vi "Notebook.vi"() -> ()   [LabVIEW 2021, in "Notebook.lvlib"]
uses:
  Notebook.lvlib
  Notebook Action Q Element.ctl
  Notebook Action List.ctl
  Notebook Parameters List.ctl
  Rich Text Box/Formatted Text.ctl
  Rich Text Box/Text Formatting.ctl
  Rich Text Box/Text Colors.ctl
  Rich Text Box/Text Style.ctl
  Rich Text Box/Text Alignment.ctl
  Notebook Theme Edit Result.ctl
  Rich Text Box/Text Format List.ctl
  GUI/3-Button Dialog Output.ctl
  Variant/Variant to Data/Variant to Boolean.vi
  Variant/Variant to Data/Variant to Path.vi
  Variant/Variant to Data/Variant to String.vi
  System.Drawing
  Rich Text Box/Rich Text Box.lvlib
  System.Windows.Forms
  Variant/Variant to Data/Variant to Data.lvlib
  Strings/Strings.lvlib
  Error/Error.lvlib
  Utilities/Utilities.lvlib
  Fits/Fits.lvlib
panel:
  in  "Text Example":refnum<k24>(container) caption="Notebook Content"
  out "Notebook Updated":bool
  out "Message":string
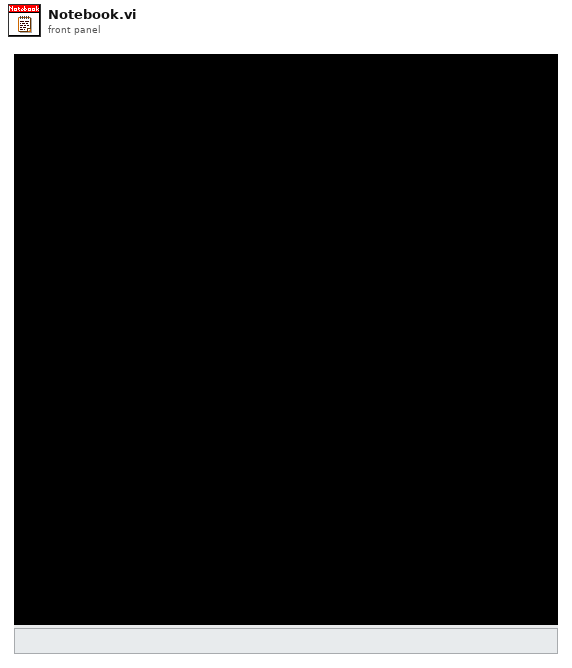
[diagram p1: front panel]
types:
  T1 = typedef "Notebook.lvlib/Notebook Parameters List.ctl" = enum16{"First Opening?", "Saved Notebook?", "Saved Notebook Path", "Beep on Error?", "Notebook Themes", "Current Theme Name"}
  T2 = enum32{"Invalid", "Standard", "Closed", "Hidden", "Minimized", "Maximized"}
  T3 = typedef "Notebook.lvlib/Notebook Action Q Element.ctl" = cluster{"Action":T4, "Variant":variant}
  T4 = typedef "Notebook.lvlib/Notebook Action List.ctl" = enum16{"Idle", "Init", "Check Content Change", "User added content", "Program added text", "Program added Picture ", "Save Notebook", "Quit", "Open", "Close", "Update Window Title", "Edit Text Styles", "Update Theme", "Save Themes", "Load Themes"}
  T5 = typedef "Rich Text Box.lvlib/Formatted Text.ctl" = cluster{"Text":string, "Text Formatting":T6}
  T6 = typedef "Rich Text Box.lvlib/Text Formatting.ctl" = cluster{"Font":string, "Text Color":T7, "Background Color":T7, "Style":T8, "Font Size":dbl, "Alignment":T9}
  T7 = typedef "Rich Text Box.lvlib/Text Colors.ctl" = enum16{"Unchanged", "Black", "Blue", "Cyan", "Maroon", "Gray", "Violet", "Green", "Light Green", "Orange", "Yellow", "Magenta", "Red", "White"}
  T8 = typedef "Rich Text Box.lvlib/Text Style.ctl" = enum16{"Regular", "Bold", "Italic", "Underline", "Strikeout"}
  T9 = typedef "Rich Text Box.lvlib/Text Alignment.ctl" = enum16{"Left", "Right", "Center"}
  T10 = typedef "Notebook.lvlib/Notebook Theme Edit Result.ctl" = enum16{"Cancelled", "Modified Theme", "New Theme", "Remove Theme"}
  T11 = typedef "Notebook.lvlib/Text Format List.ctl" = enum16{"Message", "Result", "Error", "Setting", "Verbose", "Warning"}
  T12 = typedef "Fits.lvlib/3-Button Dialog Output.ctl" = enum16{"Window Close", "Button 1", "Button 2", "Button 3"}
  T13 = typedef "Notebook.lvlib/Notebook Theme.ctl" = cluster{"Theme Name":string, "[Named Text Styles]":T14[], "Page Color":T7}
  T14 = typedef "Notebook.lvlib/Named Text Style.ctl" = cluster{"Text Formatting":T6, "Text Style Name":string}
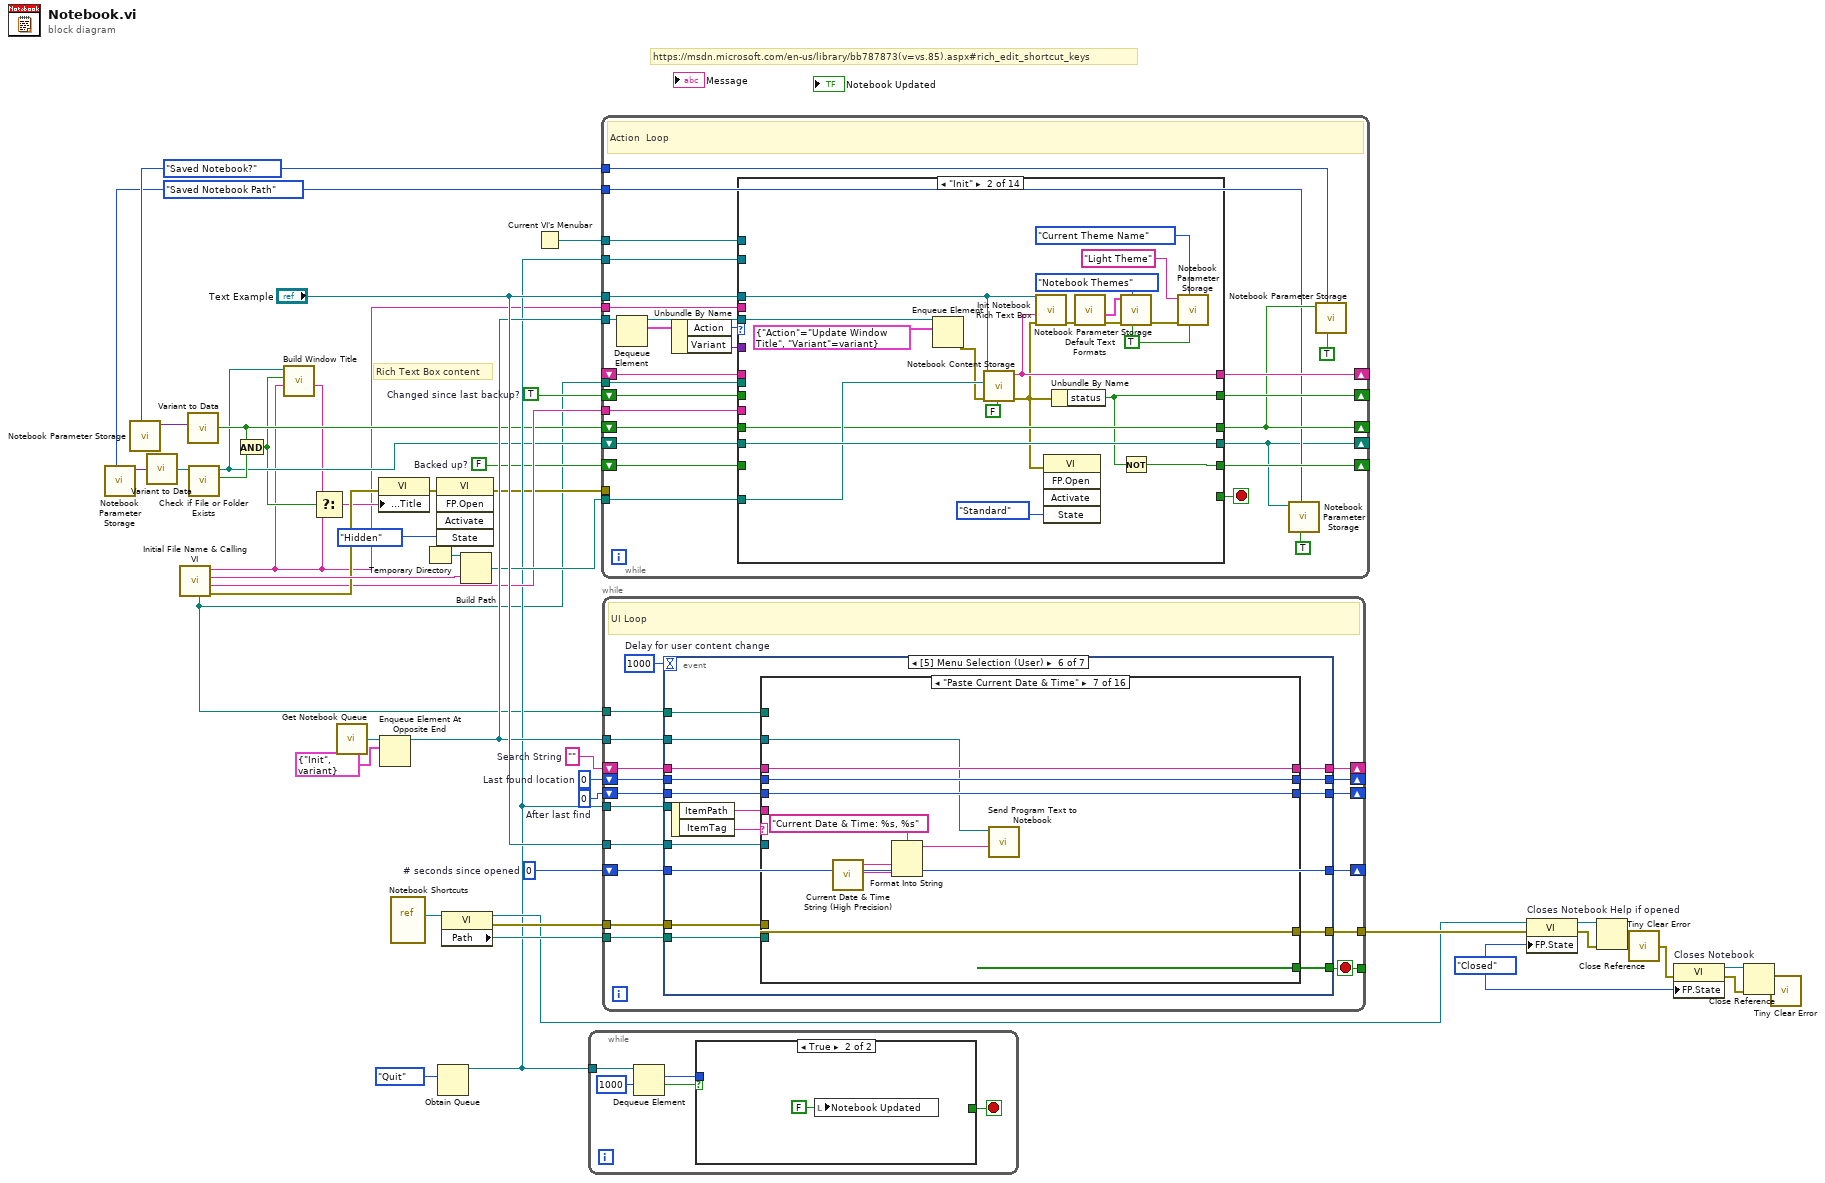
[diagram p0: block diagram]
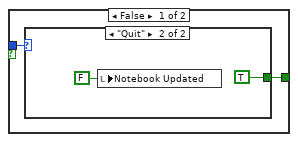
[diagram p2: hidden frame]
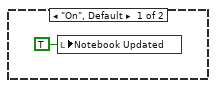
[diagram p3: hidden frame]
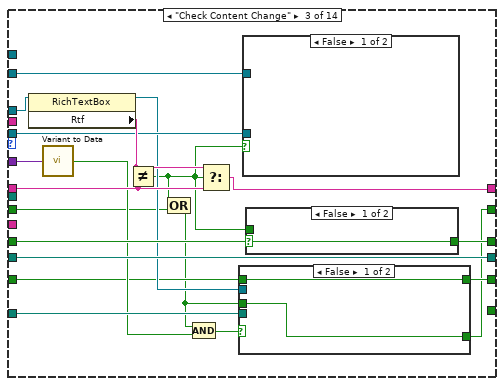
[diagram p5: hidden frame]
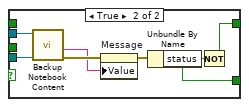
[diagram p6: hidden frame]
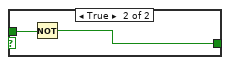
[diagram p7: hidden frame]
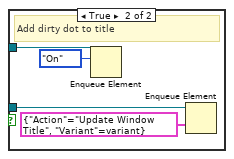
[diagram p8: hidden frame]
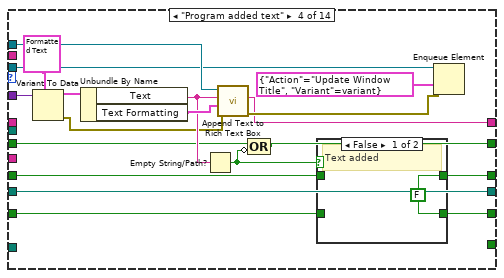
[diagram p9: hidden frame]
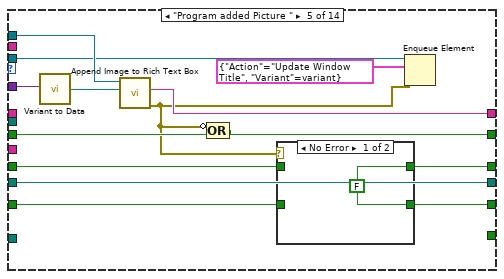
[diagram p11: hidden frame]
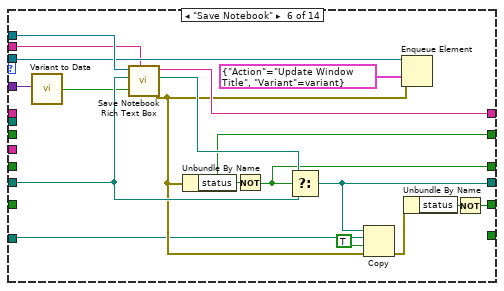
[diagram p13: hidden frame]
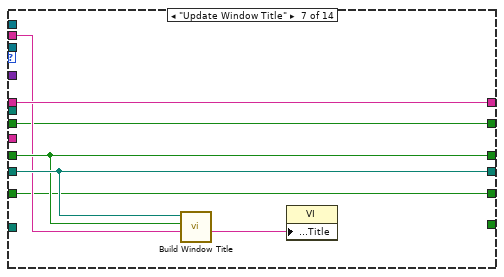
[diagram p14: hidden frame]
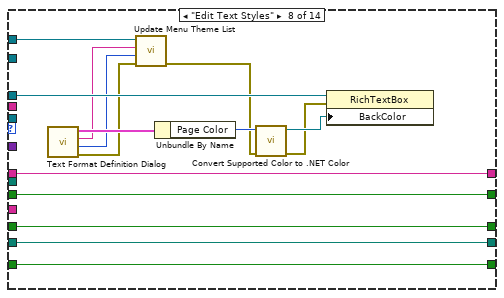
[diagram p15: hidden frame]
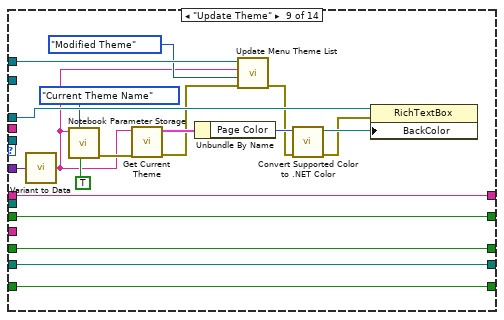
[diagram p16: hidden frame]
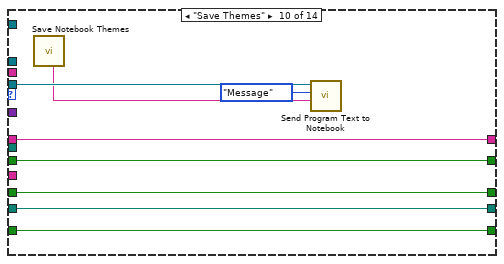
[diagram p17: hidden frame]
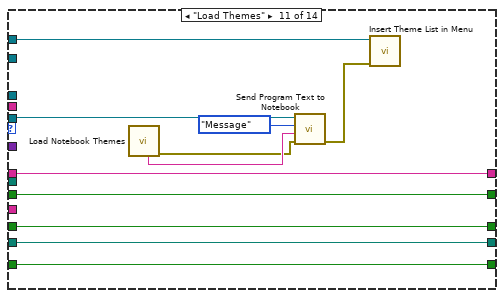
[diagram p18: hidden frame]
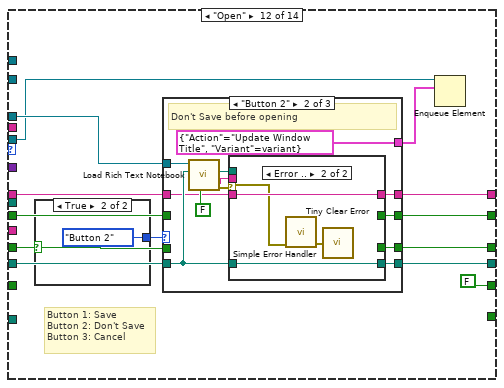
[diagram p19: hidden frame]
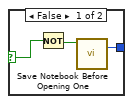
[diagram p20: hidden frame]
diagram:
  w11 = 0  # Last found location
  w12 = ""  # Search String
  w13 = 0  # After last find
  w14 = Notebook_Parameters_List."Saved Notebook Path" ("Notebook Parameter List")
  w15 = Notebook_Parameters_List."Saved Notebook?" ("Notebook Parameter List")
  w20 = TRUE  # Changed since last backup?
  w21 = FALSE  # Backed up?
  w22 = u64 0  # # seconds since opened
  w18 = T2."Closed" ("Front Panel Window:State")
  # "Rich Text Box content"
  # "https://msdn.microsoft.com/en-us/library/bb787873(v=vs.85).aspx#rich_edit_shortcut_keys"
  n1 = call "Notebook Parameter Storage.vi"("Notebook Parameter List"=w14) -> ("Data out"=w16:variant)  [unwired: 9 in, 1 out]
  n2 = call "Notebook Parameter Storage.vi"("Notebook Parameter List"=w15) -> ("Data out"=w17:variant)  [unwired: 9 in, 1 out]
  n3 = call-poly "Variant to Data.vi"("Variant"=w16) -> ("Path"=w10:path)  [unwired: 8 in]
  n4 = call "Initial File Name & Calling VI.vi"() -> ("error out"=w26:errorcluster, "Calling VI Name"=w25:string, "Backup File Name"=w40:string, "Default File Name"=w3:string, "Calling VI Path"=w2:path)  [unwired: 7 in]
  n5 = call-poly "Variant to Data.vi"("Variant"=w17) -> ("Value"=w9:bool)  [unwired: 8 in]
  n6 = call <vilib>:"Check if File or Folder Exists.vi"("path"=w10) -> ("file or folder exists?"=w8:bool, "dup path"=w6:path)  [unwired: 8 in, 1 out]
  n7 = And(x=w9, y=w8) -> (x .and. y?=w5:bool)
  n8 = call "Build Window Title.vi"("Root Window Title"=w3, "Saved Notebook?"=w5, "File Path in"=w6) -> ("Modified Window Title"=w4:string)  [unwired: 8 in]
  n9 = Select(t=w4, s=w5, f=w3) -> (s? t:f=w7:string)
  n10 = call "Get Notebook Queue.vi"() -> ("Notebook Queue"=w43:refnum<queue>)  [unwired: 9 in]
  n11 = property class="VI"(error in=w26, "Front Panel.Title"=w7) -> (error out=w38:errorcluster)  [unwired: 1 in, 1 out]
  n12 = Enqueue Element At Opposite End(queue=w43, element=T3 {"Action"=enum."Init", "Variant"=variant}) -> (queue out=w42:refnum<queue>)  [unwired: 2 in, 2 out]
  n13 = vi-ref "Notebook Shortcuts.vi"() -> (w35:refnum<vi>)
  n14 = Temporary Directory() -> (w45:path)
  n15 = invoke class="VI" method="FP.Open"(error in=w38, "State"=T2."Hidden") -> (error out=w19:errorcluster)  [unwired: 3 in, 4 out]
  n16 = Obtain Queue(element data type=enum16{"On", "Quit"}."Quit") -> (queue out=w23:refnum<queue>)  [unwired: 4 in, 2 out]
  n17 = property class="VI"(reference=w35) -> (reference out=w29:refnum<vi>, error out=w34:errorcluster, "Path"=w33:path)  [unwired: 1 in]
  n18 = Build Path(base path=w45, name or relative path=w40) -> (appended path=w39:path)
  n19 = Current VI's Menubar() -> (w1:refnum<k9>)
  n20 = while {
    tunnel: w23 -> [w52]
    stop <- w49 stop-if-true
    n21 = Dequeue Element(queue=w52, timeout in ms (-1)=1000) -> (element=w51:enum16{"On", "Quit"}, timed out?=w48:bool)  [unwired: 1 in, 2 out]
    n22 = case shown="True" w48 {
      tunnel: w51 -> [w54 _]
      tunnel: [w53 _] -> w49
      frame False {
        n23 = case shown="\"Quit\"" w54 {
          tunnel: [_ TRUE] -> w53
          frame "On", Default {
            n24 = local write "Notebook Updated"(TRUE ("Boolean Rectangle")) -> ()
          }
          frame "Quit" {
            n25 = local write "Notebook Updated"(FALSE ("Boolean Rectangle")) -> ()
          }
        }
      }
      frame True {
        n26 = local write "Notebook Updated"(FALSE ("Boolean Rectangle")) -> ()
      }
    }
  }
  n27 = while {
    tunnel: w42 -> [w85]
    shift-right: [w65] -> _
    shift-left: w9 -> [w82]
    shift-right: [w62] -> _
    shift-left: w6 -> [w81]
    tunnel: "Text Example" -> [w78]
    tunnel: w25 -> [w76]
    shift-right: [w75] -> _
    shift-left: _ -> [w74]
    tunnel: w39 -> [w73]
    tunnel: w3 -> [w72]
    tunnel: w23 -> [w71]
    shift-right: [w69] -> _
    shift-left: w21 -> [w70]
    shift-right: [w67] -> _
    shift-left: w20 -> [w68]
    tunnel: w19 -> [_]
    tunnel: w15 -> [w66]
    tunnel: w14 -> [w63]
    tunnel: w2 -> [w60]
    tunnel: w1 -> [w59]
    stop <- w77 stop-if-true
    # "Action  Loop"
    n28 = Dequeue Element(queue=w85) -> (queue out=w80:refnum<queue>, element=w84:T3)  [unwired: 2 in, 2 out]
    n29 = Unbundle By Name(w84) -> ("Action"=w83:T4, "Variant"=w79:variant)
    n30 = case shown="\"Init\"" w83 {
      tunnel: w82 -> [w90 w103 w125 w154 w174 _ w209 w226 w245 w253 w264 w271 w321 w327]
      tunnel: [w90 w103 w126 w153 w179 w195 w209 w226 w245 w253 w264 w275 w321 w327] -> w65
      tunnel: w81 -> [w89 w110 w131 w166 w183 w203 w211 w225 w244 w252 w263 w277 w322 w328]
      tunnel: [w89 w110 w131 w166 w183 w193 w211 w225 w244 w252 w263 w276 w322 w328] -> w62
      tunnel: w80 -> [_ w105 w127 w156 w177 w202 _ _ _ w248 w254 w273 w324 _]
      tunnel: w79 -> [_ _ w121 w164 w181 w200 _ _ w239 _ _ _ _ _]
      tunnel: w78 -> [_ w106 w122 w165 w182 w204 _ w221 w240 _ _ w274 w320 w338]
      tunnel: [_ _ _ _ _ _ _ _ _ _ _ _ w315 TRUE] -> w77
      tunnel: w76 -> [_ _ _ _ _ _ _ _ _ _ _ _ _ _]
      tunnel: [w88 w109 w128 w155 w176 w196 w208 w224 w243 w251 w262 w272 w323 ""] -> w75
      tunnel: w74 -> [w88 _ w129 _ _ _ w208 w224 w243 w251 w262 w269 w323 _]
      tunnel: w73 -> [_ w107 w123 _ _ w192 _ _ _ _ _ _ w319 w337]
      tunnel: w72 -> [_ _ _ _ _ w197 w207 _ _ _ _ _ _ _]
      tunnel: w71 -> [_ _ w119 _ _ _ _ _ _ _ _ _ w316 w334]
      tunnel: w70 -> [w87 _ w116 w152 w173 _ w206 w222 w241 w250 w261 _ _ _]
      tunnel: [w87 w102 w117 w151 w175 w188 w206 w222 w241 w250 w261 FALSE ("Backed up?") w312 w330] -> w69
      tunnel: w68 -> [w86 _ w114 w150 w172 _ w205 w223 w242 w249 w260 w265 w311 _]
      tunnel: [w86 w101 w113 w148 w170 w187 w205 w223 w242 w249 w260 w266 w311 FALSE ("Changed?")] -> w67
      tunnel: w60 -> [_ _ _ _ _ _ _ _ _ _ _ _ w310 _]
      tunnel: w59 -> [_ _ _ _ _ _ _ w216 w231 _ w259 _ _ _]
      frame "Idle", Default {
      }
      frame "Init" {
        w91 = TRUE ("Get(F)/Set")
        n31 = Enqueue Element(queue=w105, element=T3 {"Action"=enum."Update Window Title", "Variant"=variant}) -> (error out=w99:errorcluster)  [unwired: 2 in, 2 out]
        n32 = call "Notebook Content Storage.vi"("Save(T)/Load(F)"=FALSE ("Set(T)/Get(F)"), "Error In"=w99, "path"=w107, ".NET Refnum in"=w106) -> ("Error Out"=w100:errorcluster, "RTF content"=w109:string)  [unwired: 6 in]
        n33 = call "Init Notebook Rich Text Box.vi"("Error In"=w100, "Notebook Content"=w109, ".NET Refnum in"=w106) -> ("Error Out"=w98:errorcluster)  [unwired: 8 in]
        n34 = invoke class="VI" method="FP.Open"(error in=w100, "State"=T2."Standard") -> ()  [unwired: 3 in, 5 out]
        n35 = Unbundle By Name(w100) -> ("status"=w101:bool)
        n36 = call "Default Text Formats.vi"("Error In"=w98) -> ("Error Out"=w97:errorcluster, "Base Themes"=w96:T13[])  [unwired: 8 in, 1 out]
        n37 = call "Notebook Parameter Storage.vi"("Get(F)/Set"=w91, "Notebook Parameter List"=Notebook_Parameters_List."Notebook Themes", "Error In"=w97, "Data in"=w96) -> ("Error Out"=w94:errorcluster)  [unwired: 6 in, 1 out]
        n38 = Not(x=w101) -> (.not. x?=w102:bool)
        n39 = call "Notebook Parameter Storage.vi"("Get(F)/Set"=w91, "Notebook Parameter List"=Notebook_Parameters_List."Current Theme Name", "Error In"=w94, "Data in"="Light Theme" ("RTF content")) -> ()  [unwired: 6 in, 2 out]
      }
      frame "Check Content Change" {
        n40 = property class="RichTextBox"(reference=w122) -> (reference out=w124:refnum<k24>, "Rtf"=w130:string)  [unwired: 1 in, 1 out]
        n41 = call-poly "Variant to Data.vi"("Variant"=w121) -> ("Value"=w120:bool)  [unwired: 8 in]
        n42 = Not Equal?(x=w130, y=w129) -> (x != y?=w115:bool)
        n43 = Compound Arithmetic op=OR(w115, w114) -> (w112:bool)
        n44 = Compound Arithmetic op=AND(w112, w120) -> (w118:bool)
        n45 = Select(t=w130, s=w115, f=w129) -> (s? t:f=w128:string)
        n46 = case shown="False" w118 {
          tunnel: w124 -> [_ w140]
          tunnel: w123 -> [_ w138]
          tunnel: [w133 w135] -> w117
          tunnel: w116 -> [w133 _]
          tunnel: [w132 w134] -> w113
          tunnel: w112 -> [w132 _]
          frame False {
          }
          frame True {
            n47 = call "Backup Notebook Content.vi"("Notebook Backup Path"=w138, "Rich Text Box .NET Refnum"=w140) -> ("error out"=w139:errorcluster, "Message"=w137:string)  [unwired: 8 in]
            n48 = property on="Message" class="Str"(error in=w139, "Value"=w137) -> (error out=w136:errorcluster)  [unwired: 1 in, 1 out]
            n49 = Unbundle By Name(w136) -> ("status"=w134:bool)
            n50 = Not(x=w134) -> (.not. x?=w135:bool)
          }
        }
        n51 = case shown="False" w115 {
          tunnel: w127 -> [_ w147]
          tunnel: w119 -> [_ w145]
          frame False {
          }
          frame True {
            # "Add dirty dot to title"
            n52 = Enqueue Element(queue=w145, element=enum16{"On", "Quit"}."On") -> ()  [unwired: 2 in, 3 out]
            n53 = Enqueue Element(queue=w147, element=T3 {"Action"=enum."Update Window Title", "Variant"=variant}) -> ()  [unwired: 2 in, 3 out]
          }
        }
        n54 = case shown="False" w125 {
          selector: w125 -> [w141 _]
          tunnel: w115 -> [_ w143]
          tunnel: [w141 w142] -> w126
          frame False {
          }
          frame True {
            n55 = Not(x=w143) -> (.not. x?=w142:bool)
          }
        }
      }
      frame "Program added text" {
        n56 = Variant To Data(type=T5 {"Text"="", "Text Formatting"={"Font"="", "Text Color"=enum."Unchanged", "Background Color"=enum."Unchanged", "Style"=enum."Regular", "Font Size"=-1.0, "Alignment"=enum."Left"}} ("Formatted Text"), Variant=w164) -> (data=w162:T5, error out=w159:errorcluster)  [unwired: 1 in]
        n57 = Unbundle By Name(w162) -> ("Text"=w160:string, "Text Formatting"=w161:T6)
        n58 = Empty String/Path?(string/path=w160) -> (empty?=w149:bool)
        n59 = call "Append Text to Rich Text Box.vi"("error in (no error)"=w159, "Text Formatting"=w161, "String"=w160, ".NET Refnum in"=w165) -> ("Error Out"=w157:errorcluster, "Rtf Content"=w155:string)  [unwired: 5 in, 1 out]
        n60 = Compound Arithmetic op=OR(w150, invert w149) -> (w148:bool)
        n61 = case shown="False" w149 {
          tunnel: w154 -> [_ w169]
          tunnel: [w167 w169] -> w153
          tunnel: w152 -> [_ w168]
          tunnel: [w167 w168] -> w151
          frame False {
            w167 = FALSE ("Saved Notebook?")
            # "Text added"
          }
          frame True {
            # "No change"
          }
        }
        n62 = Enqueue Element(queue=w156, element=T3 {"Action"=enum."Update Window Title", "Variant"=variant}, error in (no error)=w157) -> ()  [unwired: 1 in, 3 out]
      }
      frame "Program added Picture " {
        n63 = call-poly "Variant to Data.vi"("Variant"=w181) -> ("Path"=w180:path)  [unwired: 8 in]
        n64 = call "Append Image to Rich Text Box.vi"("Image File Path"=w180, ".NET Refnum in"=w182) -> ("error out"=w171:errorcluster, "Rtf Content"=w176:string)  [unwired: 8 in]
        n65 = Compound Arithmetic op=OR(invert w171, w172) -> (w170:bool)
        n66 = case shown="No Error" w171 {
          tunnel: [w184 w186] -> w179
          tunnel: [w184 w185] -> w175
          tunnel: w174 -> [_ w186]
          tunnel: w173 -> [_ w185]
          frame No Error {
            w184 = FALSE ("Saved?")
          }
          frame Error {
          }
        }
        n67 = Enqueue Element(queue=w177, element=T3 {"Action"=enum."Update Window Title", "Variant"=variant}, error in (no error)=w171) -> ()  [unwired: 1 in, 3 out]
      }
      frame "Save Notebook" {
        n68 = call-poly "Variant to Data.vi"("Variant"=w200) -> ("Value"=w199:bool)  [unwired: 8 in]
        n69 = call "Save Notebook Rich Text Box.vi"("Default Notebook File Name (Notebook)"=w197, "Dialog (F)"=w199, "File Path Control"=w203, ".NET Refnum in"=w204) -> ("Error Out"=w194:errorcluster, "File Path out"=w198:path, "Rtf Content"=w196:string)  [unwired: 4 in, 1 out]
        n70 = Unbundle By Name(w194) -> ("status"=w187:bool)
        n71 = Not(x=w187) -> (.not. x?=w195:bool)
        n72 = Select(t=w198, s=w195, f=w203) -> (s? t:f=w193:path)
        n73 = Copy(8:w194, 9:TRUE ("overwrite (F)"), 10:w192, 11:w193) -> (0:w190:errorcluster)  [unwired: 1 in, 2 out]
        n74 = Enqueue Element(queue=w202, element=T3 {"Action"=enum."Update Window Title", "Variant"=variant}, error in (no error)=w194) -> ()  [unwired: 1 in, 3 out]
        n75 = Unbundle By Name(w190) -> ("status"=w189:bool)
        n76 = Not(x=w189) -> (.not. x?=w188:bool)
      }
      frame "Update Window Title" {
        n77 = call "Build Window Title.vi"("Root Window Title"=w207, "Saved Notebook?"=w209, "File Path in"=w211) -> ("Modified Window Title"=w210:string)  [unwired: 8 in]
        n78 = property class="VI"("Front Panel.Title"=w210) -> ()  [unwired: 2 in, 2 out]
      }
      frame "Edit Text Styles" {
        n79 = call "Text Format Definition Dialog.vi"() -> ("Error Out"=w213:errorcluster, "Result"=w215:T10, "Theme Name"=w214:string, "Notebook Theme"=w218:T13)  [unwired: 8 in]
        n80 = call "Update Menu Theme List.vi"("error in (no error)"=w213, "Result"=w215, "Theme Name"=w214, "Menu in"=w216) -> ("error out"=w212:errorcluster)  [unwired: 7 in]
        n81 = Unbundle By Name(w218) -> ("Page Color"=w217:T7)
        n82 = call "Convert Supported Color to .NET Color.vi"("error in (no error)"=w212, "Text Color"=w217) -> ("error out"=w219:errorcluster, ".NET Color"=w220:refnum<k24>)  [unwired: 8 in]
        n83 = property class="RichTextBox"(reference=w221, error in=w219, "BackColor"=w220) -> ()  [unwired: 2 out]
      }
      frame "Update Theme" {
        n84 = call-poly "Variant to Data.vi"("Variant"=w239) -> ("String"=w229:string)  [unwired: 8 in]
        n85 = call "Notebook Parameter Storage.vi"("Get(F)/Set"=TRUE, "Notebook Parameter List"=Notebook_Parameters_List."Current Theme Name", "Data in"=w229) -> ("Error Out"=w233:errorcluster)  [unwired: 7 in, 1 out]
        n86 = call "Get Current Theme.vi"("Error In"=w233, "Theme Name"=w229) -> ("Error Out"=w228:errorcluster, "Notebook Theme"=w232:T13)  [unwired: 7 in, 1 out]
        n87 = Unbundle By Name(w232) -> ("Page Color"=w236:T7)
        n88 = call "Update Menu Theme List.vi"("error in (no error)"=w228, "Result"=Notebook_Theme_Edit_Result."Modified Theme", "Theme Name"=w229, "Menu in"=w231) -> ("error out"=w227:errorcluster)  [unwired: 7 in]
        n89 = call "Convert Supported Color to .NET Color.vi"("error in (no error)"=w227, "Text Color"=w236) -> ("error out"=w237:errorcluster, ".NET Color"=w238:refnum<k24>)  [unwired: 8 in]
        n90 = property class="RichTextBox"(reference=w240, error in=w237, "BackColor"=w238) -> ()  [unwired: 2 out]
      }
      frame "Save Themes" {
        n91 = call "Save Notebook Themes.vi"() -> ("Message"=w247:string)  [unwired: 8 in, 3 out]
        n92 = call "Send Program Text to Notebook.vi"("Text (none)"=w247, "Text Format (Message)"=Text_Format_List."Message" ("Text Format"), "Notebook Queue in"=w248) -> ()  [unwired: 8 in, 1 out]
      }
      frame "Load Themes" {
        n93 = call "Load Notebook Themes.vi"() -> ("error out"=w256:errorcluster, "Message"=w257:string)  [unwired: 8 in, 2 out]
        n94 = call "Send Program Text to Notebook.vi"("Error In"=w256, "Text (none)"=w257, "Text Format (Message)"=Text_Format_List."Message" ("Text Format"), "Notebook Queue in"=w254) -> ("Error Out"=w255:errorcluster)  [unwired: 7 in]
        n95 = call "Insert Theme List in Menu.vi"("error in (no error)"=w255, "Menu in"=w259) -> ()  [unwired: 9 in, 1 out]
      }
      frame "Open" {
        # "Button 1: Save\nButton 2: Don't Save\nButton 3: Cancel"
        n96 = case shown="True" w271 {
          selector: w271 -> [w280 _]
          tunnel: [w279 3-Button_Dialog_Output."Button 2" ("Save/Don't Save/Cancel")] -> w270
          frame False {
            n97 = Not(x=w280) -> (.not. x?=w278:bool)
            n98 = call "Save Notebook Before Opening One.vi"("Not saved?"=w278) -> ("Save/Don't Save/Cancel"=w279:T12)  [unwired: 9 in, 1 out]
          }
          frame True {
          }
        }
        n99 = case shown="\"Button 2\"" w270 {
          tunnel: w277 -> [w285 w293 w308]
          tunnel: [w285 w298 w308] -> w276
          tunnel: [w286 w292 w307] -> w275
          tunnel: w271 -> [w286 _ w307]
          tunnel: w274 -> [_ w297 _]
          tunnel: [w284 w288 w309] -> w272
          tunnel: w269 -> [w284 w289 w309]
          tunnel: [T3 {"Action"=enum."Save Notebook", "Variant"=variant} ("element") T3 {"Action"=enum."Update Window Title", "Variant"=variant} ("element") _] -> w268
          tunnel: [w282 w287 w306] -> w266
          tunnel: w265 -> [w282 _ w306]
          frame "Button 1" {
            # "Save"
            # "Save"
          }
          frame "Button 2" {
            # "Don't Save before opening"
            n100 = call "Load Rich Text Notebook.vi"("Backup?"=FALSE, "File Path Control"=w293, ".NET Refnum in"=w297) -> ("Error Out"=w290:errorcluster, "File Path out"=w296:path, "RTF content"=w291:string)  [unwired: 4 in, 2 out]
            n101 = case shown="Error .." w290 {
              selector: w290 -> [_ w303]
              tunnel: [w301 w305] -> w298
              tunnel: w296 -> [w301 _]
              tunnel: w293 -> [_ w305]
              tunnel: [w299 _] -> w292
              tunnel: w291 -> [w300 _]
              tunnel: w289 -> [_ w304]
              tunnel: [w300 w304] -> w288
              tunnel: [w299 _] -> w287
              frame No Error {
                w299 = TRUE ("status")
              }
              frame Error {
                n102 = call <vilib>:"Simple Error Handler.vi"("error in (no error)"=w303) -> ("error out"=w302:errorcluster)  [unwired: 4 in, 4 out]
                n103 = call "Tiny Clear Error.vi"("Error In"=w302) -> ()  [unwired: 8 in, 1 out]
              }
            }
          }
          frame "Button 3", Default {
            # "Cancel"
          }
        }
        n104 = Enqueue Element(queue=w273, element=w268) -> ()  [unwired: 2 in, 3 out]
      }
      frame "Close" {
        n105 = call "Close Notebook Window Action.vi"("Notebook Saved?"=w321, "Main VI Path"=w310, "Notebook Queue"=w324) -> ("Quit?"=w315:bool)  [unwired: 8 in]
        n106 = call "Backup Notebook Content.vi"("Notebook Backup Path"=w319, "Rich Text Box .NET Refnum"=w320) -> ("error out"=w317:errorcluster, "Message"=w318:string)  [unwired: 8 in]
        n107 = case shown="True" w315 {
          tunnel: w316 -> [_ w325]
          frame False {
          }
          frame True {
            n108 = Enqueue Element(queue=w325, element=enum16{"On", "Quit"}."Quit") -> ()  [unwired: 2 in, 3 out]
          }
        }
        n109 = property on="Message" class="Str"(error in=w317, "Value"=w318) -> (error out=w314:errorcluster)  [unwired: 1 in, 1 out]
        n110 = Unbundle By Name(w314) -> ("status"=w313:bool)
        n111 = Not(x=w313) -> (.not. x?=w312:bool)
      }
      frame "Quit" {
        n112 = Enqueue Element(queue=w334, element=enum16{"On", "Quit"}."Quit") -> ()  [unwired: 2 in, 3 out]
        n113 = call "Backup Notebook Content.vi"("Notebook Backup Path"=w337, "Rich Text Box .NET Refnum"=w338) -> ("error out"=w335:errorcluster, "Message"=w336:string)  [unwired: 8 in]
        n114 = property on="Message" class="Str"(error in=w335, "Value"=w336) -> (error out=w332:errorcluster)  [unwired: 1 in, 1 out]
        n115 = Unbundle By Name(w332) -> ("status"=w331:bool)
        n116 = Not(x=w331) -> (.not. x?=w330:bool)
      }
    }
    n117 = call "Notebook Parameter Storage.vi"("Get(F)/Set"=TRUE, "Notebook Parameter List"=w63, "Data in"=w62) -> ()  [unwired: 7 in, 2 out]
    n118 = call "Notebook Parameter Storage.vi"("Get(F)/Set"=TRUE, "Notebook Parameter List"=w66, "Data in"=w65) -> ()  [unwired: 7 in, 2 out]
  }
  n119 = while {
    tunnel: w42 -> [w357]
    tunnel: "Text Example" -> [w355]
    tunnel: w34 -> [w354]
    tunnel: w33 -> [w353]
    tunnel: [w352] -> _
    tunnel: [w351] -> w30
    tunnel: w23 -> [w350]
    shift-right: [w348] -> _
    shift-left: w22 -> [w349]
    shift-right: [w347] -> _
    shift-left: w13 -> [w344]
    shift-right: [w346] -> _
    shift-left: w12 -> [w345]
    shift-right: [w342] -> _
    shift-left: w11 -> [w343]
    tunnel: w2 -> [w341]
    stop <- w352 stop-if-true
    w356 = 1000  # Delay for user content change
    # "UI Loop"
    n120 = event shown="[5] Menu Selection (User)" {
      selector: _ -> [_ _ _ _ _ _ _]
      dyn-events: _ -> [_ _ _ _ _ _ _]
      timeout: w356 -> [_ _ _ _ _ _ _]
      tunnel: [w366 _ _ _ _ w493 _] -> w352
      tunnel: w357 -> [w368 w374 w455 _ w479 w494 _]
      tunnel: w355 -> [_ w378 _ w463 _ w488 w636]
      tunnel: w341 -> [w358 _ _ _ _ w481 _]
      tunnel: w354 -> [_ _ _ _ _ w492 _]
      tunnel: w353 -> [_ _ _ _ _ w491 _]
      tunnel: [_ _ _ _ _ w490 _] -> w351
      tunnel: w350 -> [_ w373 _ _ _ _ _]
      tunnel: w349 -> [w365 w372 w454 w465 w476 w489 w635]
      tunnel: [w365 w372 w454 w465 w474 w489 w635] -> w348
      tunnel: [w360 w370 w452 w458 w470 w487 w633] -> w347
      tunnel: [w361 w371 w453 w459 w471 w486 w634] -> w346
      tunnel: w345 -> [w361 w371 w453 w459 w471 w485 w634]
      tunnel: w344 -> [w360 w370 w452 w458 w470 w484 w633]
      tunnel: w343 -> [w359 w369 w451 w457 w469 w482 w632]
      tunnel: [w359 w369 w451 w457 w469 w483 w632] -> w342
      event Panel Close? {
        n121 = event-data() -> ()  [unwired: 1 in, 1 out]
        n122 = call "Notebook Parameter Storage.vi"("Notebook Parameter List"=Notebook_Parameters_List."Saved Notebook?") -> ("Data out"=w364:variant)  [unwired: 9 in, 1 out]
        n123 = call-poly "Variant to Data.vi"("Variant"=w364) -> ("Value"=w362:bool)  [unwired: 8 in]
        n124 = call "Close Notebook Window Action.vi"("Notebook Saved?"=w362, "Main VI Path"=w358, "Notebook Queue"=w368) -> ("Quit?"=w366:bool)  [unwired: 8 in]
        n125 = event-data("Discard?"=TRUE) -> ()  [unwired: 1 in, 1 out]
      }
      event "Text Example": Shortcut Menu Selection (User) {
        n126 = event-data() -> ("ItemTag"=w379:string)  [unwired: 1 in]
        n127 = property class="RichTextBox"(reference=w378) -> (reference out=w375:refnum<k24>, error out=w376:errorcluster, "SelectionFont"=w377:refnum<k24>)  [unwired: 1 in]
        n128 = case shown="\"B_Black\", \"B_Blue\", \"B_Cyan\", \"B_Gray\", \"B_Green\", \"B_Light Green\", \"B_Magenta\", \"B_Maroon\", \"B_Orange\", \"B_Red\", \"B_Violet\", \"B_White\", \"B_Yellow\"" w379 {
          selector: w379 -> [_ w390 w397 w411 w432]
          tunnel: w377 -> [_ w384 w401 _ _]
          tunnel: w376 -> [_ w383 w396 w412 w434]
          tunnel: w375 -> [_ w380 w393 w413 w435]
          tunnel: w374 -> [_ _ _ _ _]
          tunnel: w373 -> [_ _ w391 w409 w433]
          frame "" {
          }
          frame "5 pt", Default {
            n129 = property class="Font"(reference=w384, error in=w383) -> (error out=w387:errorcluster, "Name"=w388:string, "Style"=w382:i32)  [unwired: 1 out]
            n130 = Scan From String(format string="%d pt", input string=w390) -> (output 1=w381:i32)  [unwired: 3 in, 3 out]
            n131 = constructor class="Font"(error in=w387, "familyName"=w388, "emSize"=w381, "unit"=w382) -> (reference out=w385:refnum<k24>, error out=w386:errorcluster)  [unwired: 2 in, 4 out]
            n132 = property class="RichTextBox"(reference=w380, error in=w386, "SelectionFont"=w385) -> ()  [unwired: 2 out]
          }
          frame "Bold", "Italic", "Regular", "Strikeout", "Underline" {
            n133 = disable-structure shown="Disabled" {
              disable-tunnel: w391 -> [w402 _]
              frame Disabled {
                n134 = Enqueue Element(queue=w402, element=enum16{"On", "Quit"}."On") -> ()  [unwired: 2 in, 3 out]
              }
              frame Enabled {
              }
            }
            n135 = property class="Font"(reference=w401, error in=w396) -> (error out=w395:errorcluster, "Name"=w400:string, "SizeInPoints"=w399:sgl)  [unwired: 1 out]
            n136 = case shown="\"Bold\"" w397 {
              tunnel: [w404 w405 w406 w407 w408] -> w398
              frame "Regular", Default {
                w404 = 0 items=["Regular"=0, "Bold"=1, "Italic"=2, "Underline"=4, "Strikeout"=8] ("style")
              }
              frame "Bold" {
                w405 = 1 items=["Regular"=0, "Bold"=1, "Italic"=2, "Underline"=4, "Strikeout"=8] ("style")
              }
              frame "Italic" {
                w406 = 2 items=["Regular"=0, "Bold"=1, "Italic"=2, "Underline"=4, "Strikeout"=8] ("style")
              }
              frame "Underline" {
                w407 = 4 items=["Regular"=0, "Bold"=1, "Italic"=2, "Underline"=4, "Strikeout"=8] ("style")
              }
              frame "Strikeout" {
                w408 = 8 items=["Regular"=0, "Bold"=1, "Italic"=2, "Underline"=4, "Strikeout"=8] ("style")
              }
            }
            n137 = constructor class="Font"(error in=w395, "familyName"=w400, "emSize"=w399, "unit"=w398) -> (reference out=w392:refnum<k24>, error out=w394:errorcluster)  [unwired: 2 in, 4 out]
            n138 = property class="RichTextBox"(reference=w393, error in=w394, "SelectionFont"=w392) -> ()  [unwired: 2 out]
          }
          frame "Black", "Blue", "Cyan", "Gray", "Green", "Light Green", "Magenta", "Maroon", "Orange", "Red", "Violet", "White", "Yellow" {
            n139 = case shown="\"Orange\"" w411 {
              tunnel: [Text_Colors."Black" ("Text Color") Text_Colors."Blue" ("Text Color") Text_Colors."Cyan" ("Text Color") Text_Colors."Gray" ("Text Color") Text_Colors."Green" ("Text Color") Text_Colors."Light Green" ("Text Color") Text_Colors."Magenta" ("Text Color") Text_Colors."Maroon" ("Text Color") Text_Colors."Orange" ("Text Color") Text_Colors."Red" ("Text Color") Text_Colors."Violet" ("Text Color") Text_Colors."White" ("Text Color") Text_Colors."Yellow" ("Text Color")] -> w410
              frame "Black", Default {
              }
              frame "Blue" {
              }
              frame "Cyan" {
              }
              frame "Gray" {
              }
              frame "Green" {
              }
              frame "Light Green" {
              }
              frame "Magenta" {
              }
              frame "Maroon" {
              }
              frame "Orange" {
              }
              frame "Red" {
              }
              frame "Violet" {
              }
              frame "White" {
              }
              frame "Yellow" {
              }
            }
            n140 = disable-structure shown="Disabled" {
              disable-tunnel: w409 -> [w414 _]
              frame Disabled {
                n141 = Enqueue Element(queue=w414, element=enum16{"On", "Quit"}."On") -> ()  [unwired: 2 in, 3 out]
              }
              frame Enabled {
              }
            }
            n142 = call "Set RTB Selection Text Color.vi"("Error In"=w412, "Text Color"=w410, ".NET RTB Refnum in"=w413) -> ()  [unwired: 7 in, 2 out]
          }
          frame "B_Black", "B_Blue", "B_Cyan", "B_Gray", "B_Green", "B_Light Green", "B_Magenta", "B_Maroon", "B_Orange", "B_Red", "B_Violet", "B_White", "B_Yellow" {
            n143 = disable-structure shown="Disabled" {
              disable-tunnel: w433 -> [w450 _]
              frame Disabled {
                n144 = Enqueue Element(queue=w450, element=enum16{"On", "Quit"}."On") -> ()  [unwired: 2 in, 3 out]
              }
              frame Enabled {
              }
            }
            n145 = String Subset(string=w432, offset (0)=2) -> (substring=w430:string)  [unwired: 1 in]
            n146 = case shown="\"Cyan\"" w430 {
              tunnel: [Text_Colors."Black" ("Text Color") Text_Colors."Blue" ("Text Color") Text_Colors."Cyan" ("Text Color") Text_Colors."Gray" ("Text Color") Text_Colors."Green" ("Text Color") Text_Colors."Light Green" ("Text Color") Text_Colors."Magenta" ("Text Color") Text_Colors."Maroon" ("Text Color") Text_Colors."Orange" ("Text Color") Text_Colors."Red" ("Text Color") Text_Colors."Violet" ("Text Color") Text_Colors."White" ("Text Color") Text_Colors."Yellow" ("Text Color")] -> w431
              frame "Black", Default {
              }
              frame "Blue" {
              }
              frame "Cyan" {
              }
              frame "Gray" {
              }
              frame "Green" {
              }
              frame "Light Green" {
              }
              frame "Magenta" {
              }
              frame "Maroon" {
              }
              frame "Orange" {
              }
              frame "Red" {
              }
              frame "Violet" {
              }
              frame "White" {
              }
              frame "Yellow" {
              }
            }
            n147 = call "Set RTB Selection Text Background Color.vi"("Error In"=w434, "Text Background Color"=w431, ".NET RTB Refnum in"=w435) -> ()  [unwired: 7 in, 2 out]
          }
        }
      }
      event "Text Example": Value Change {
        n148 = event-data() -> ()  [unwired: 1 in, 3 out]
        n149 = Enqueue Element(queue=w455, element=T3 {"Action"=enum."Check Content Change", "Variant"=variant}) -> ()  [unwired: 2 in, 3 out]
      }
      event "Text Example": Mouse Down? {
        n150 = event-data() -> ("Button"=w460:u16, "Coords.Horizontal"=w462:i32, "Coords.Vertical"=w461:i32)  [unwired: 1 in]
        n151 = case shown="1" w460 {
          tunnel: w463 -> [_ w468]
          tunnel: w462 -> [_ w467]
          tunnel: w461 -> [_ w466]
          frame 2, Default {
            # "right click"
          }
          frame 1 {
            # "Left Click"
            n152 = call "Set Cursor to Mouse Click.vi"("Vertical"=w466, "Horizontal"=w467, "RichTextBox Refnum"=w468) -> ()  [unwired: 8 in, 1 out]
          }
        }
        n153 = event-data("Discard?"=FALSE) -> ()  [unwired: 4 in, 1 out]
      }
      event Timeout {
        w475 = u64 300  # Delay for backup (x timeout)
        n154 = event-data() -> ()  [unwired: 1 in, 1 out]
        n155 = Increment(x=w476) -> (x+1=w474:u64)
        n156 = Quotient & Remainder(x=w474, y=w475) -> (x-y*floor(x/y)=w473:u64)  [unwired: 1 out]
        n157 = Equal To 0?(x=w473) -> (x = 0?=w472:bool)
        n158 = Bundle By Name(cluster=T3 {"Action"=enum."Check Content Change", "Variant"=variant} ("element"), "Variant"=w472) -> (w477:T3)
        n159 = Enqueue Element(queue=w479, element=w477) -> ()  [unwired: 2 in, 3 out]
      }
      event Menu Selection (User) {
        n160 = event-data() -> ("ItemPath"=w480:string, "ItemTag"=w495:string)  [unwired: 1 in]
        n161 = case shown="\"Paste Current Date & Time\"" w495 {
          selector: w495 -> [_ _ _ _ _ _ _ _ _ _ _ _ w603 w613 _ _]
          tunnel: w494 -> [_ w505 w513 w521 w531 _ w536 _ _ _ _ w594 w604 w615 _ _]
          tunnel: [_ _ _ _ w530 _ _ _ _ _ _ _ _ _ _ _] -> w493
          tunnel: w481 -> [_ _ _ _ w529 _ _ _ _ _ _ _ _ _ _ _]
          tunnel: w492 -> [w499 w503 w509 w517 w528 w535 w541 w550 w560 w580 w593 w599 w608 w619 w625 w630]
          tunnel: w491 -> [_ _ _ _ _ _ _ _ _ _ _ _ _ _ _ w631]
          tunnel: [w499 w503 w509 w517 w528 w535 w541 w548 w556 w572 w593 w599 w608 w619 w625 w629] -> w490
          tunnel: w488 -> [_ _ _ _ _ _ _ w549 w561 w581 _ _ _ _ _ _]
          tunnel: [w497 w501 w507 w515 w523 w533 w539 w546 w558 w573 w592 w598 w607 w618 w623 w627] -> w487
          tunnel: [w498 w502 w508 w516 w524 w534 w540 w547 w555 w571 w591 w597 w606 w617 w624 w628] -> w486
          tunnel: w485 -> [w498 w502 w508 w516 w524 w534 w540 _ w555 w571 w591 w597 w606 w617 w624 w628]
          tunnel: w484 -> [w497 w501 w507 w515 w523 w533 w539 _ w559 _ w592 w598 w607 w618 w623 w627]
          tunnel: [w496 w500 w506 w514 w522 w532 w538 w545 w553 w575 w590 w596 w605 w616 w622 w626] -> w483
          tunnel: w482 -> [w496 w500 w506 w514 w522 w532 w538 _ _ w579 w590 w596 w605 w616 w622 w626]
          tunnel: w480 -> [_ _ _ _ _ _ _ _ _ _ _ _ w602 _ _ _]
          frame "---------File----------" {
          }
          frame "Open" {
            n162 = Enqueue Element(queue=w505, element=T3 {"Action"=enum."Open", "Variant"=variant}) -> ()  [unwired: 2 in, 3 out]
          }
          frame "Save" {
            w510 = FALSE  # No dialog
            n163 = Bundle By Name(cluster=T3 {"Action"=enum."Save Notebook", "Variant"=variant} ("element"), "Variant"=w510) -> (w511:T3)
            n164 = Enqueue Element(queue=w513, element=w511) -> ()  [unwired: 2 in, 3 out]
          }
          frame "Save As..." {
            w518 = TRUE  # Dialog
            n165 = Bundle By Name(cluster=T3 {"Action"=enum."Save Notebook", "Variant"=variant} ("element"), "Variant"=w518) -> (w519:T3)
            n166 = Enqueue Element(queue=w521, element=w519) -> ()  [unwired: 2 in, 3 out]
          }
          frame "Close" {
            n167 = call "Notebook Parameter Storage.vi"("Notebook Parameter List"=Notebook_Parameters_List."Saved Notebook?") -> ("Data out"=w527:variant)  [unwired: 9 in, 1 out]
            n168 = call-poly "Variant to Data.vi"("Variant"=w527) -> ("Value"=w526:bool)  [unwired: 8 in]
            n169 = call "Close Notebook Window Action.vi"("Notebook Saved?"=w526, "Main VI Path"=w529, "Notebook Queue"=w531) -> ("Quit?"=w530:bool)  [unwired: 8 in]
          }
          frame "----------Edit----------" {
          }
          frame "Paste Current Date & Time" {
            n170 = call "Current Date & Time String (High Precision).vi"() -> ("time string"=w542:string, "date string"=w543:string)  [unwired: 8 in, 2 out]
            n171 = Format Into String(format string="Current Date & Time: %s, %s" ("initial string"), w543, w542) -> (resulting string=w537:string)  [unwired: 2 in, 1 out]
            n172 = call "Send Program Text to Notebook.vi"("Text (none)"=w537, "Notebook Queue in"=w536) -> ()  [unwired: 9 in, 1 out]
          }
          frame "Find..." {
            n173 = call "Notebook Find String.vi"("error in (no error)"=w550, ".NET Refnum in"=w549) -> ("error out"=w548:errorcluster, "String location"=w545:i32, "String to search for:"=w547:string, "Location after string"=w546:i32)  [unwired: 5 in, 1 out]
          }
          frame "Find Next" {
            n174 = call "Notebook Find String after.vi"("error in (no error)"=w560, "After position"=w559, "Search String"=w555, ".NET Refnum in"=w561) -> ("error out"=w557:errorcluster, "Location after string"=w551:i32, "String location"=w552:i32, ".NET Refnum out"=w554:refnum<k24>)  [unwired: 4 in]
            n175 = case shown="Error" w557 {
              selector: w557 -> [w562 _]
              tunnel: [w564 w565] -> w558
              tunnel: [w562 w569] -> w556
              tunnel: w555 -> [_ w568]
              tunnel: w554 -> [_ w567]
              tunnel: [w563 w566] -> w553
              tunnel: w552 -> [w563 _]
              tunnel: w551 -> [w564 _]
              frame No Error {
              }
              frame Error {
                # "if end, restart from start"
                n176 = call "Notebook Find String after.vi"("Search String"=w568, ".NET Refnum in"=w567) -> ("error out"=w569:errorcluster, "Location after string"=w565:i32, "String location"=w566:i32)  [unwired: 6 in, 1 out]
              }
            }
          }
          frame "Find Previous" {
            n177 = Decrement(x=w579) -> (x-1=w578:i32)
            n178 = call "Notebook Find String before.vi"("error in (no error)"=w580, "Before position"=w578, "Search String"=w571, ".NET Refnum in"=w581) -> ("error out"=w577:errorcluster, "Location after string"=w574:i32, "String location"=w576:i32, ".NET Refnum out"=w570:refnum<k24>)  [unwired: 4 in]
            n179 = case shown="Error .." w577 {
              selector: w577 -> [w582 _]
              tunnel: w576 -> [w584 _]
              tunnel: [w584 w588] -> w575
              tunnel: w574 -> [w583 _]
              tunnel: [w583 w588] -> w573
              tunnel: [w582 w589] -> w572
              tunnel: w571 -> [_ w587]
              tunnel: w570 -> [_ w586]
              frame No Error {
              }
              frame Error {
                # "if beginning reached, start from end"
                n180 = call "Notebook Find String before.vi"("Before position"=2147483647, "Search String"=w587, ".NET Refnum in"=w586) -> ("error out"=w589:errorcluster, "Location after string"=w588:i32)  [unwired: 5 in, 2 out]
              }
            }
          }
          frame "---- Styles ----" {
          }
          frame "Edit Text Styles" {
            n181 = Enqueue Element(queue=w594, element=T3 {"Action"=enum."Edit Text Styles", "Variant"=variant}) -> ()  [unwired: 2 in, 3 out]
          }
          frame "Dark Theme", "Light Theme", Default {
            n182 = Search and Replace String(input string=w602, search string="Styles") -> (number of replacements=w600:i32)  [unwired: 6 in, 3 out]
            n183 = case shown="1, Default" w600 {
              tunnel: w604 -> [_ w611]
              tunnel: w603 -> [_ w609]
              frame 0 {
              }
              frame 1, Default {
                n184 = Bundle By Name(cluster=T3 {"Action"=enum."Update Theme", "Variant"=variant} ("element"), "Variant"=w609) -> (w610:T3)
                n185 = Enqueue Element(queue=w611, element=w610) -> ()  [unwired: 2 in, 3 out]
              }
            }
          }
          frame "Load Themes", "Save Themes" {
            n186 = case shown="\"Save Themes\"" w613 {
              tunnel: [T3 {"Action"=enum."Save Themes", "Variant"=variant} ("element") T3 {"Action"=enum."Load Themes", "Variant"=variant} ("element") _] -> w614
              frame "Save Themes" {
              }
              frame "Load Themes" {
              }
              frame Default {
              }
            }
            n187 = Enqueue Element(queue=w615, element=w614) -> ()  [unwired: 2 in, 3 out]
          }
          frame "-------- Help ---------" {
          }
          frame "Show Notebook Shortcuts" {
            n188 = call "Run Vi.vi"("VI Path"=w631, "error in (no error)"=w630) -> ("error out"=w629:errorcluster)  [unwired: 6 in, 1 out]
          }
        }
      }
      event Panel Resize {
        n189 = event-data() -> ()  [unwired: 1 in, 1 out]
        n190 = disable-structure shown="Disabled" {
          disable-tunnel: w636 -> [w637 _]
          frame Disabled {
            n191 = invoke class="RichTextBox" method="ScrollToCaret"(reference=w637) -> ()  [unwired: 2 in, 3 out]
          }
          frame Enabled {
          }
        }
      }
    }
  }
  n192 = property on="Closes Notebook Help if opened" class="VI"(reference=w29, error in=w30, "FP.State"=w18) -> (reference out=w31:refnum<vi>, error out=w32:errorcluster)
  n193 = Close Reference(reference=w31, error in (no error)=w32) -> (error out=w28:errorcluster)
  n194 = call "Tiny Clear Error.vi"("Error In"=w28) -> ("no Error Out"=w27:errorcluster)  [unwired: 8 in]
  n195 = property on="Closes Notebook" class="VI"(error in=w27, "FP.State"=w18) -> (reference out=w47:refnum<vi>, error out=w37:errorcluster)  [unwired: 1 in]
  n196 = Close Reference(reference=w47, error in (no error)=w37) -> (error out=w36:errorcluster)
  n197 = call "Tiny Clear Error.vi"("Error In"=w36) -> ()  [unwired: 8 in, 1 out]
